vi "set_ButtonLabels.vi"(0 "HB_Dialog in":refnum<class "HB_Dialog.lvclass">, 7 "T button name (\"OK\")":string="OK", 9 "F button name (\"Cancel\")":string="Cancel", 11 "error in (no error)":errorcluster) -> (4 "HB_Dialog out":refnum<class "HB_Dialog.lvclass">, 15 "error out":errorcluster)   [LabVIEW 2009, in "HB_Inherance_Example.lvlib" / "HB_Dialog.lvclass"]
doc: "Set button label text."
uses:
  HB_Dialog.lvclass
  HB_Dialog.lvclass/HB_Dialog.ctl
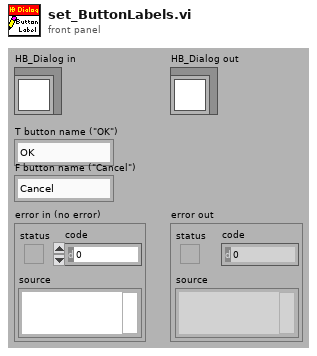
[diagram p1: front panel]
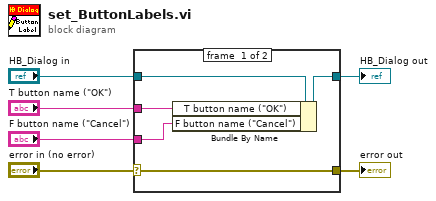
[diagram p0: block diagram]
diagram:
  n1 = case shown="No Error" "error in (no error)" {
    selector: "error in (no error)" -> [w11 w12]
    tunnel: [w11 w12] -> w5
    tunnel: [w9 w13] -> w3
    tunnel: "HB_Dialog in" -> [w10 w13]
    tunnel: "T button name (\"OK\")" -> [w8 _]
    tunnel: "F button name (\"Cancel\")" -> [w7 _]
    frame #0 {
      n2 = Bundle By Name(cluster=w10, "T button name (\"OK\")"=w8, "F button name (\"Cancel\")"=w7) -> (w9:refnum<class "HB_Dialog.lvclass">)
    }
    frame #1 {
    }
  }
  "error out" <- w5
  "HB_Dialog out" <- w3
